vi "LineWidthFilter.vi"(0 "Image Pixels (U8) 2":u8[][](array[numeric]), 1 "X Min":i32=4, 2 "X max":i32=22) -> (3 "Image Pixels (U8)":u8[][](array[numeric]))   [LabVIEW 2009]
panel:
  out "Waveform Graph":u8[](graph)
  out "Waveform Graph 2":u8[](graph)
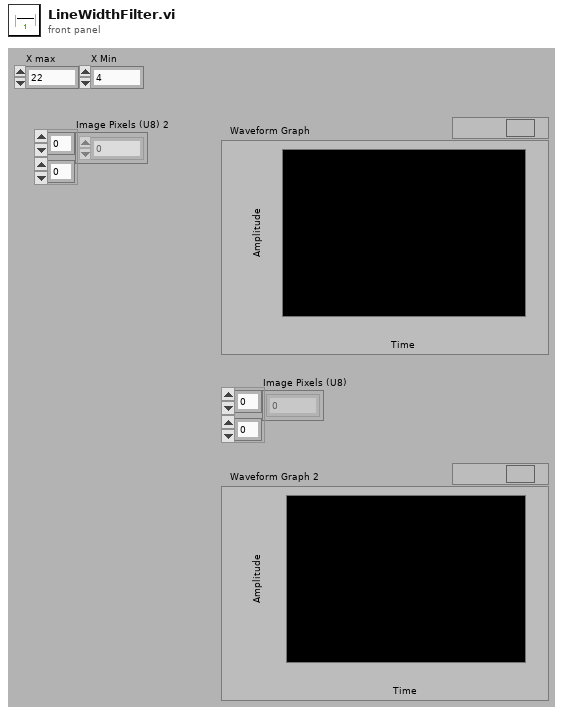
[diagram p1: front panel]
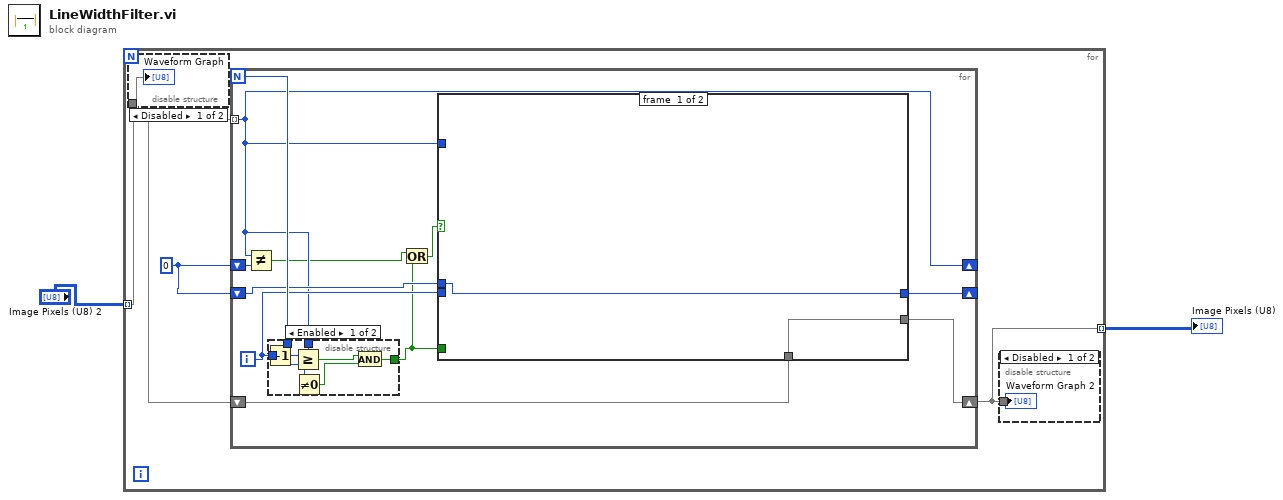
[diagram p0: block diagram]
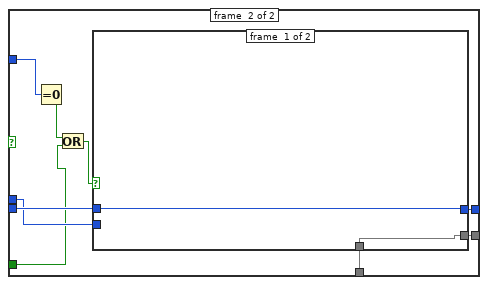
[diagram p4: hidden frame]
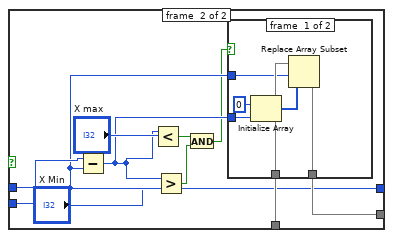
[diagram p5: hidden frame]
diagram:
  n1 = for {
    tunnel: "Image Pixels (U8) 2" -> [w4] mode=indexing
    tunnel: [w3] -> w2 mode=indexing
    w5 = u8 0
    n2 = disable-structure shown="Disabled" {
      disable-tunnel: w4 -> [w6 _]
      frame #0 {
        "Waveform Graph" <- w6
      }
      frame #1 {
      }
    }
    n3 = for {
      N -> [w14]
      tunnel: w4 -> [w11] mode=indexing
      shift-right: [w11] -> _
      shift-left: w5 -> [w18]
      shift-right: [w17] -> _
      shift-left: w5 -> [w12]
      shift-right: [w15] -> w3
      shift-left: w4 -> [w16]
      i -> [w13]
      n4 = Not Equal?(x=w11, y=w18) -> (x != y?=w10:bool)
      n5 = disable-structure shown="Enabled" {
        disable-tunnel: w13 -> [w55 _]
        disable-tunnel: w14 -> [w51 _]
        disable-tunnel: [w50 _] -> w9
        disable-tunnel: w11 -> [w49 _]
        frame #0 {
          n6 = Increment(x=w55) -> (x+1=w54:i32)
          n7 = Greater Or Equal?(x=w54, y=w51) -> (x >= y?=w53:bool)
          n8 = Not Equal To 0?(x=w49) -> (x != 0?=w52:bool)
          n9 = And(x=w53, y=w52) -> (x .and. y?=w50:bool)
        }
        frame #1 {
        }
      }
      n10 = Or(x=w10, y=w9) -> (x .or. y?=w8:bool)
      n11 = case shown="True" w8 {
        tunnel: [w19 w29] -> w17
        tunnel: w16 -> [w20 w28]
        tunnel: [w20 w27] -> w15
        tunnel: w13 -> [_ w26]
        tunnel: w12 -> [w19 w25]
        tunnel: w11 -> [_ w24]
        tunnel: w9 -> [_ w22]
        frame #0 {
        }
        frame #1 {
          n12 = Equal To 0?(x=w24) -> (x = 0?=w23:bool)
          n13 = Or(x=w23, y=w22) -> (x .or. y?=w21:bool)
          n14 = case shown="True" w21 {
            tunnel: [w30 w38] -> w29
            tunnel: w26 -> [w30 w41]
            tunnel: w25 -> [_ w38]
            tunnel: w28 -> [w31 w40]
            tunnel: [w31 w39] -> w27
            frame #0 {
            }
            frame #1 {
              n15 = Subtract(x=w41, y=w38) -> (x-y=w35:i32)
              n16 = Less?(x=w35, y="X max") -> (x < y?=w34:bool)
              n17 = Greater?(x=w35, y="X Min") -> (0:w33:bool)
              n18 = And(x=w34, y=w33) -> (x .and. y?=w32:bool)
              n19 = case shown="False" w32 {
                tunnel: w40 -> [w47 w48]
                tunnel: w35 -> [w46 _]
                tunnel: w38 -> [w43 _]
                tunnel: [w42 w48] -> w39
                frame #0 {
                  n20 = Initialize Array(u8 0 ("element"), w46) -> (w44:u8[])
                  n21 = Replace Array Subset(array=w47, new element=w44, index=w43) -> (w42:u8[])
                }
                frame #1 {
                }
              }
            }
          }
        }
      }
    }
    n22 = disable-structure shown="Disabled" {
      disable-tunnel: w3 -> [w7 _]
      frame #0 {
        "Waveform Graph 2" <- w7
      }
      frame #1 {
      }
    }
  }
  "Image Pixels (U8)" <- w2
